vi "Set Label.vi"(8 "Error In":errorcluster, 9 "Label":string, 10 "UID":i32, 11 "Controls":variant) -> (0 "Error Out":errorcluster, 3 "Controls":variant)   [LabVIEW 2014]
uses:
  Control Info.ctl
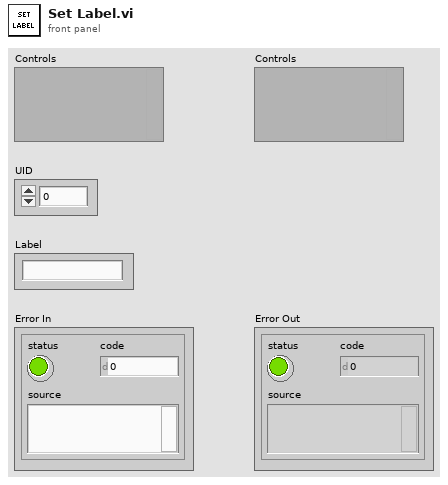
[diagram p1: front panel]
types:
  T1 = typedef "Control Info.ctl" = cluster{"Label":string, "Description":string}
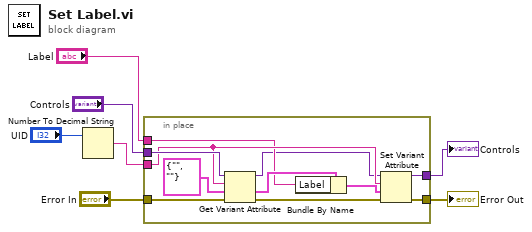
[diagram p0: block diagram]
diagram:
  n1 = Number To Decimal String(number="UID") -> (decimal integer string=w3:string)  [unwired: 1 in]
  n2 = in-place {
    in-place-border: "Controls" -> [w18]
    in-place-border: w3 -> [w17]
    in-place-border: "Label" -> [w14]
    in-place-border: [w10] -> w5
    in-place-border: [w9] -> w6
    in-place-border: "Error In" -> [w8]
    n3 = Get Variant Attribute(Variant=w18, name=w17, default value (empty Variant)=T1 {"Label"="", "Description"=""} ("Control Info"), error in=w8) -> (duplicate Variant=w11:variant, value=w15:T1, error out=w12:errorcluster)  [unwired: 1 out]
    n4 = Bundle By Name(cluster=w15, "Label"=w14) -> (w13:T1)
    n5 = Set Variant Attribute(Variant=w11, name=w17, value=w13, error in=w12) -> (Variant out=w10:variant, error out=w9:errorcluster)  [unwired: 1 out]
  }
  "Controls" <- w5
  "Error Out" <- w6
